vi "Configure Output Frequency.vi"(0 "VISA resource name":refnum<visa-resource-name>, 1 "Output Frequency Slew Rate (9.9E+37 Hz)":dbl=9.9e+37 format="%#.4g", 2 "Output Frequency Slew Mode (0: Fix)":u16(ring) items=["Fixed", "Step", "Pulse", "List"], 5 "Output Frequency (60 Hz)":dbl=60.0 format="%#.4g", 7 "Output Frequency Mode (0: Fixed)":u16(ring) items=["Fixed", "Step", "Pulse", "List"], 11 "error in (no error)":errorcluster, 12 "Triggered Output Frequency (60.0 Hz)":dbl=60.0 format="%#.4g", 13 "Triggered Output Frequency Slew Rate (9.9E+37 Hz)":dbl=9.9e+37 format="%#.4g") -> (4 "VISA resource name out":refnum<visa-resource-name>, 15 "error out":errorcluster)   [LabVIEW 2020, in "Agilent 681x Series.lvlib"]
doc: "Configures the output frequency and frequency slew rate settings of the instrument."
uses:
  <instrlib>/Agilent 681x Series/Agilent 681x Series.lvlib
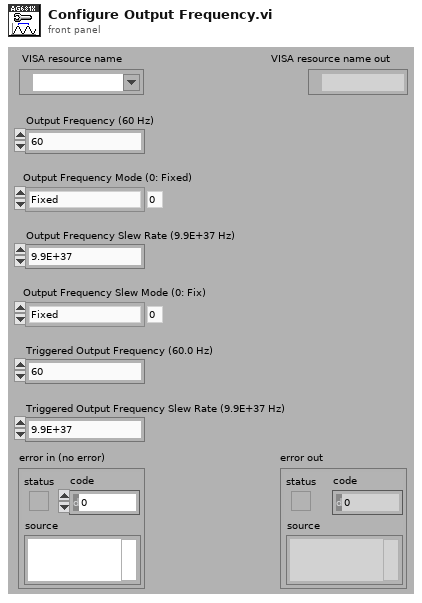
[diagram p1: front panel]
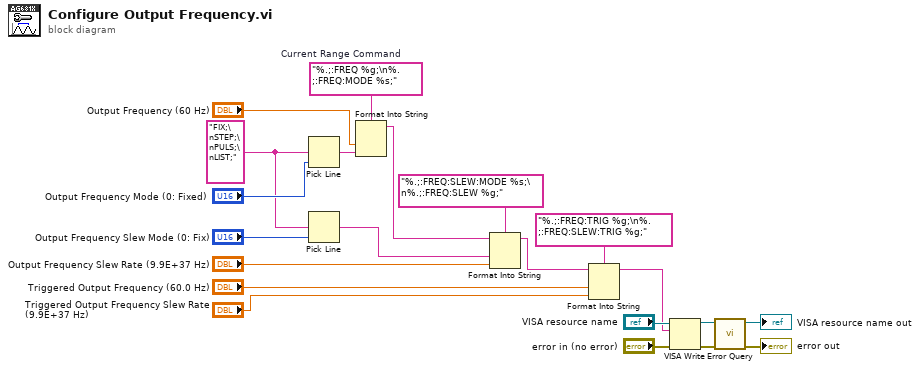
[diagram p0: block diagram]
diagram:
  w11 = "FIX;\nSTEP;\nPULS;\nLIST;" ("multi-line string")
  w17 = "%.;:FREQ %g;\n%.;:FREQ:MODE %s;"  # Current Range Command
  n1 = Pick Line(multi-line string=w11, line index="Output Frequency Mode (0: Fixed)") -> (output string=w12:string)  [unwired: 1 in]
  n2 = Pick Line(multi-line string=w11, line index="Output Frequency Slew Mode (0: Fix)") -> (output string=w9:string)  [unwired: 1 in]
  n3 = Format Into String(format string=w17, "Output Frequency (60 Hz)", w12) -> (resulting string=w7:string)  [unwired: 2 in, 1 out]
  n4 = Format Into String(format string="%.;:FREQ:SLEW:MODE %s;\n%.;:FREQ:SLEW %g;", initial string=w7, w9, "Output Frequency Slew Rate (9.9E+37 Hz)") -> (resulting string=w4:string)  [unwired: 1 in, 1 out]
  n5 = Format Into String(format string="%.;:FREQ:TRIG %g;\n%.;:FREQ:SLEW:TRIG %g;", initial string=w4, "Triggered Output Frequency (60.0 Hz)", "Triggered Output Frequency Slew Rate (9.9E+37 Hz)") -> (resulting string=w2:string)  [unwired: 1 in, 1 out]
  n6 = VISA Write(VISA resource name="VISA resource name", write buffer=w2, error in (no error)="error in (no error)") -> (VISA resource name out=w19:refnum<visa-resource-name>, error out=w18:errorcluster)  [unwired: 1 out]
  n7 = call <instrlib>:"Error Query.vi"("error in (no error)"=w18, "VISA resource name"=w19) -> ("error out"=→"error out":errorcluster, "VISA resource name out"=→"VISA resource name out":refnum<visa-resource-name>)  [unwired: 6 in, 2 out]
